vi "Result_Test.vi"(8 "error in (no error)":errorcluster caption="entrée d'erreur (pas d'erreur)", 11 "Get_Voltage en entrée":refnum<class "Zigbee_Net_Leave.lvclass">) -> (0 "error out":errorcluster caption="sortie d'erreur", 3 "Get_Voltage en sortie":refnum<class "Zigbee_Net_Leave.lvclass">)   [LabVIEW 2020, in "Library Test.lvlib" / "Zigbee_Net_Leave.lvclass"]
uses:
  Zigbee_Net_Leave.lvclass
  C:/Users/ngarcin/OneDrive - Altyor/Standard TB/Class/Test/Test (Default)/Test (Default).lvclass
  C:/Users/ngarcin/OneDrive - Altyor/Standard TB/Class/Test/Zigbee_Send_Command_UART/Zigbee_Send_Command_UART.lvclass
  Zigbee_Send_Command_UART/Zigbee_Send_Command_UART.lvclass
  Zigbee_Net_Leave.lvclass/Zigbee_Net_Leave.ctl
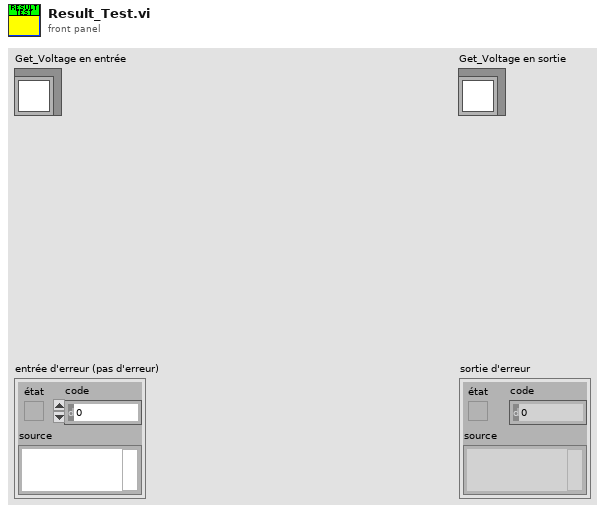
[diagram p1: front panel]
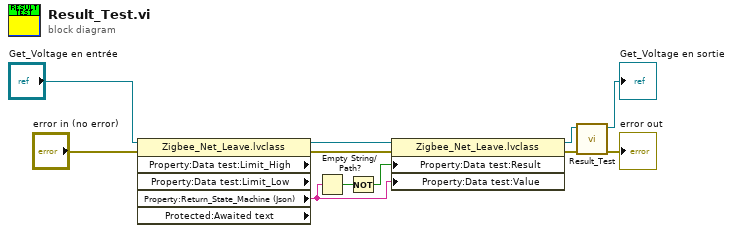
[diagram p0: block diagram]
diagram:
  n1 = property class="Zigbee_Net_Leave.lvclass" props=["Property:Data test:Limit_High", "Property:Data test:Limit_Low", "Property:Return_State_Machine (Json)", "Protected:Awaited text"](reference="Get_Voltage en entrée", error in="error in (no error)") -> (reference out=w9:refnum<class "Zigbee_Net_Leave.lvclass">, error out=w8:errorcluster, "Property:Return_State_Machine (Json)"=w1:string)  [unwired: 3 out]
  n2 = Empty String/Path?(string/path=w1) -> (empty?=w3:bool)
  n3 = Not(x=w3) -> (.not. x?=w2:bool)
  n4 = property class="Zigbee_Net_Leave.lvclass"(reference=w9, error in=w8, "Property:Data test:Result"=w2, "Property:Data test:Value"=w1) -> (reference out=w4:refnum<class "Zigbee_Net_Leave.lvclass">, error out=w5:errorcluster)
  n5 = call-parent "Result_Test.vi"("error in (no error)"=w5, "Get_Voltage en entrée"=w4) -> ("error out"=→"error out":errorcluster, "Get_Voltage en sortie"=→"Get_Voltage en sortie":refnum<class "Zigbee_Net_Leave.lvclass">)  [unwired: 8 in]
